vi "StopSignal-TestMain4.vi"() -> ()   [LabVIEW 2017]
uses:
  StopSignal.lvlib
panel:
  out "timestamp #1":timestamp
  out "timestamp #3":timestamp
  out "timestamp #4":timestamp
  out "reason #4":string
  out "reason #1":string
  out "reason #3":string
  out "current time":timestamp
  in  "stop":bool
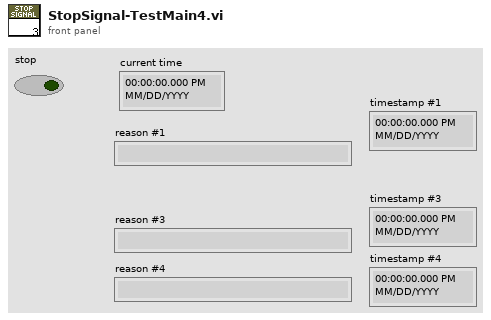
[diagram p1: front panel]
types:
  T1 = typedef "StopSignal.lvlib/StopSignal.ctl" = refnum<k1>
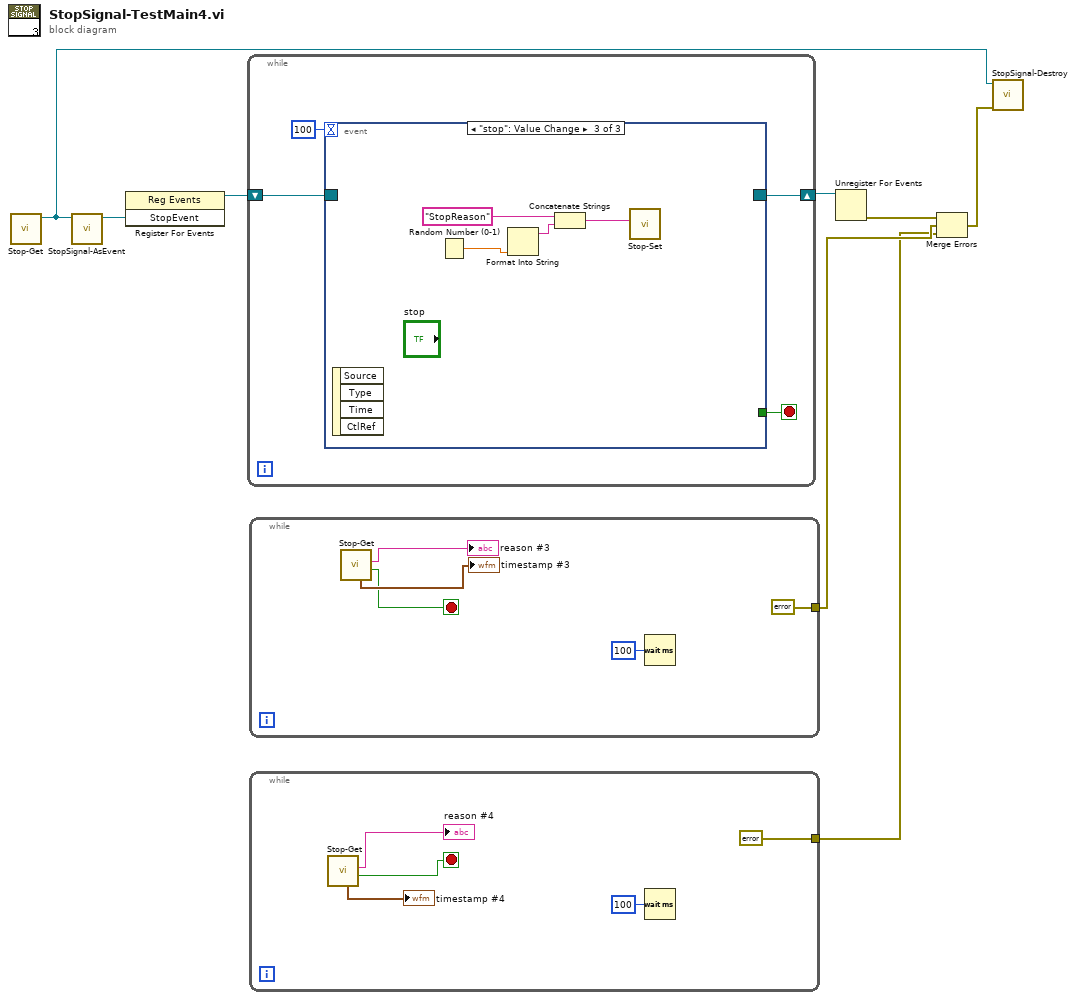
[diagram p0: block diagram]
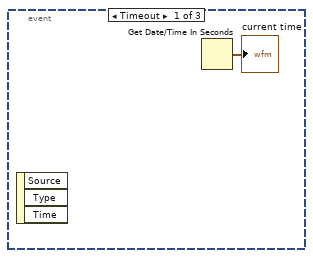
[diagram p2: hidden frame]
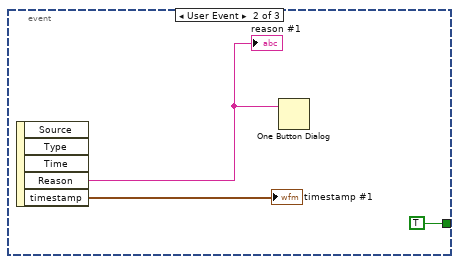
[diagram p3: hidden frame]
diagram:
  n1 = call "Stop-Get.vi"() -> ("StopSignal"=w1:T1)  [unwired: 7 in, 4 out]
  n2 = call "StopSignal-AsEvent.vi"("StopSignal"=w1) -> ("StopEvent"=w5:refnum<user-event>)  [unwired: 9 in, 1 out]
  n3 = register-events(w5) -> (reference out=w8:refnum<event-registration>)  [unwired: 2 in, 1 out]
  n4 = while {
    shift-right: [w9] -> w7
    shift-left: w8 -> [w12]
    stop <- w11 stop-if-true
    n5 = event shown="[2] \"stop\": Value Change" {
      selector: w12 -> [_ _ _]
      dyn-events: [_ _ _] -> w9
      timeout: 100 -> [_ _ _]
      tunnel: [_ TRUE _] -> w11
      event Timeout {
        n6 = event-data() -> ()  [unwired: 1 in, 3 out]
        n7 = Get Date/Time In Seconds() -> (seconds since 1Jan1904=→"current time":timestamp)
      }
      event User Event {
        n8 = event-data() -> ("Reason"=w15:string, "timestamp"=→"timestamp #1":timestamp)  [unwired: 1 in, 3 out]
        "reason #1" <- w15
        n9 = One Button Dialog(message=w15) -> ()  [unwired: 1 in, 1 out]
      }
      event "stop": Value Change {
        n10 = event-data() -> ()  [unwired: 1 in, 4 out]
        n11 = Random Number (0-1)() -> (number: 0 to 1=w19:dbl)
        n12 = Format Into String(w19) -> (resulting string=w18:string)  [unwired: 3 in, 1 out]
        n13 = Concatenate Strings("StopReason" ("event data"), w18) -> (w17:string)
        n14 = call "Stop-Set.vi"("Reason"=w17) -> ()  [unwired: 10 in, 1 out]
      }
    }
  }
  n15 = while {
    tunnel: [errorcluster {"status"=FALSE, "code"=0, "source"=""} ("error out")] -> w3
    stop <- w21 stop-if-true
    n16 = call "Stop-Get.vi"() -> ("Stop?"=w21:bool, "Reason"=→"reason #3":string, "timestamp"=→"timestamp #3":timestamp)  [unwired: 7 in, 2 out]
    n17 = Wait (ms)(milliseconds to wait=u32 100) -> ()  [unwired: 1 out]
  }
  n18 = while {
    tunnel: [errorcluster {"status"=FALSE, "code"=0, "source"=""} ("error out")] -> w2
    stop <- w28 stop-if-true
    n19 = call "Stop-Get.vi"() -> ("Stop?"=w28:bool, "Reason"=→"reason #4":string, "timestamp"=→"timestamp #4":timestamp)  [unwired: 7 in, 2 out]
    n20 = Wait (ms)(milliseconds to wait=u32 100) -> ()  [unwired: 1 out]
  }
  n21 = Unregister For Events(event registration refnum=w7) -> (error out=w6:errorcluster)  [unwired: 1 in]
  n22 = Merge Errors(w6, w3, w2) -> (w4:errorcluster)
  n23 = call "StopSignal-Destroy.vi"("error in (no error)"=w4, "StopSignal"=w1) -> ()  [unwired: 8 in, 2 out]
